vi "Parser signal by dbc.vi"(5 "ID array":i32[](array[numeric]) format="%.0x", 7 "NameShort":string[][](array[string])=[["Radar_AK_AMP", "Radar_AK_ANG", "Radar_AK_BSD_FLG", "Radar_AK_DST", "Radar_AK_ELE", "Radar_AK_EXST_PRB", "Radar_AK_Ego_Car_SPD", "Radar_AK_ID", "Radar_AK_LNG_ACC", "Radar_AK_MOV_FLG", "Radar_AK_RESERVE", "Radar_AK_SPD", "Radar_AK_Vx", "Radar_AK_Vy", "Radar_AK_Vz", "", "", "", "", "", "", "", "", "", "", "", "", "", "", ""], ["Radar_BK_2_AMP", "Radar_BK_2_ANG", "Radar_BK_2_DST", "Radar_BK_2_ELE", "Radar_BK_2_SPD", "Radar_BK_3_AMP", "Radar_BK_3_ANG", "Radar_BK_3_DST", "Radar_BK_3_ELE", "Radar_BK_3_SPD", "Radar_BK_4_AMP", "Radar_BK_4_ANG", "Radar_BK_4_DST", "Radar_BK_4_ELE", "Radar_BK_4_SPD", "Radar_BK_5_AMP", "Radar_BK_5_ANG", "Radar_BK_5_DST", "Radar_BK_5_ELE", "Radar_BK_5_SPD", "Radar_BK_6_AMP", "Radar_BK_6_ANG", "Radar_BK_6_DST", "Radar_BK_6_ELE", "Radar_BK_6_SPD", "Radar_BK_AMP", "Radar_BK_ANG", "Radar_BK_DST", "Radar_BK_ELE", "Radar_BK_SPD"], ["Radar_Header_Cdi_Number", "Radar_Header_Frame_Peroid", "Radar_Header_Frame_Type", "Radar_Header_Frame_id", "Radar_Header_Raw_Number", "Radar_Header_Track_Output_Number", "", "", "", "", "", "", "", "", "", "", "", "", "", "", "", "", "", "", "", "", "", "", "", ""], ["Radar_AK_Header_Number", "Radar_AK_Run_Time", "", "", "", "", "", "", "", "", "", "", "", "", "", "", "", "", "", "", "", "", "", "", "", "", "", "", "", ""]], 8 "error in (no error)":errorcluster caption="错误输入（无错误）", 9 "payload":u8[](array[numeric])=[140, 5, 0, 0, 0, 205, 218, 172, 202, 134, 212, 0, 0, 0, 0, 0, 20, 6, 0, 0, 0, 205, 214, 171, 199, 128, 12, 0, 0, 0, 0, 0, 107, 6, 0, 0, 0, 205, 86, 79, 7, 253, 54, 0, 0, 0, 0, 0, 0, 0, 0, 0, 0, 0, 0, 0, 0, 0, 0, 0, 0, 0, 0, 0] format="%.0x", 10 "ID":u32=1024 format="%.0x", 11 "Session":refnum<k21>[](array[refnum])) -> (0 "error out":errorcluster caption="错误输出", 1 "signal data":dbl[](array[numeric])=[1.0, -0.87, 0.0, 0.0, 0.27, 0.0, 0.0, 0.0, 0.0, -101.0, 14.200000000000001, 0.0, 27.32, -74.0, 0.0, 1.0, 0.25, 0.0, 0.0, 0.03, 0.0, 0.0, 0.0, 0.0, -101.0, 15.56, 0.0, 19.63, -82.0, 0.0, 0.0, 1.09, 0.0, 0.0, -0.12, 0.0, 0.0, 0.0, 0.0, -101.0, 16.43, 0.0, 18.71, -82.0, 0.0, 0.0, 0.0, 0.0, 0.0, 0.0, 0.0, 0.0, 0.0, 0.0, -255.0, 0.0, 0.0, 0.0, -255.0, 0.0] format="%.2f", 2 "Names":string[](array[string])=["LGU1_azAmb", "LGU1_azAngle", "LGU1_azAngleQly", "LGU1_elAmb", "LGU1_elAngle", "LGU1_elAngleQly", "LGU1_existProb", "LGU1_locPeerIdx", "LGU1_measStatus", "LGU1_noi", "LGU1_radDist", "LGU1_radVel", "LGU1_rcsEst", "LGU1_sigPwr", "LGU1_velQly", "LGU2_azAmb", "LGU2_azAngle", "LGU2_azAngleQly", "LGU2_elAmb", "LGU2_elAngle", "LGU2_elAngleQly", "LGU2_existProb", "LGU2_locPeerIdx", "LGU2_measStatus", "LGU2_noi", "LGU2_radDist", "LGU2_radVel", "LGU2_rcsEst", "LGU2_sigPwr", "LGU2_velQly", "LGU3_azAmb", "LGU3_azAngle", "LGU3_azAngleQly", "LGU3_elAmb", "LGU3_elAngle", "LGU3_elAngleQly", "LGU3_existProb", "LGU3_locPeerIdx", "LGU3_measStatus", "LGU3_noi", "LGU3_radDist", "LGU3_radVel", "LGU3_rcsEst", "LGU3_sigPwr", "LGU3_velQly", "LGU4_azAmb", "LGU4_azAngle", "LGU4_azAngleQly", "LGU4_elAmb", "LGU4_elAngle", "LGU4_elAngleQly", "LGU4_existProb", "LGU4_locPeerIdx", "LGU4_measStatus", "LGU4_noi", "LGU4_radDist", "LGU4_radVel", "LGU4_rcsEst", "LGU4_sigPwr", "LGU4_velQly"])   [LabVIEW 2024]
uses:
  <vilib>/xnet/xnet.llb/XNET Frame CAN.ctl
  <vilib>/xnet/xnet.llb/XNET Frame Type CAN.ctl
  <vilib>/xnet/xnet.llb/XNET Convert (Frame CAN to Signal).vi
panel:
  out "time":u32=4
  in  "frame data":T1[](array[typedef])=[{"timestamp"=timestamp(0 s since 1904-01-01), "payload"=[], "identifier"=0, "type"=16, "extended?"=FALSE, "echo?"=FALSE}] {"payload" format="%x"; "timestamp" format="%<%.7X\n%x>T"; "type" items=["CAN Data"=0, "CAN Remote"=1, "CAN Bus Error"=2, "CAN 2.0 Data"=8, "CAN FD Data"=16, "CAN FD+BRS Data"=24, "J1939 Data"=192, "Delay"=224, "Log Trigger"=225, "Start Trigger"=226]; "identifier" format="%x"}
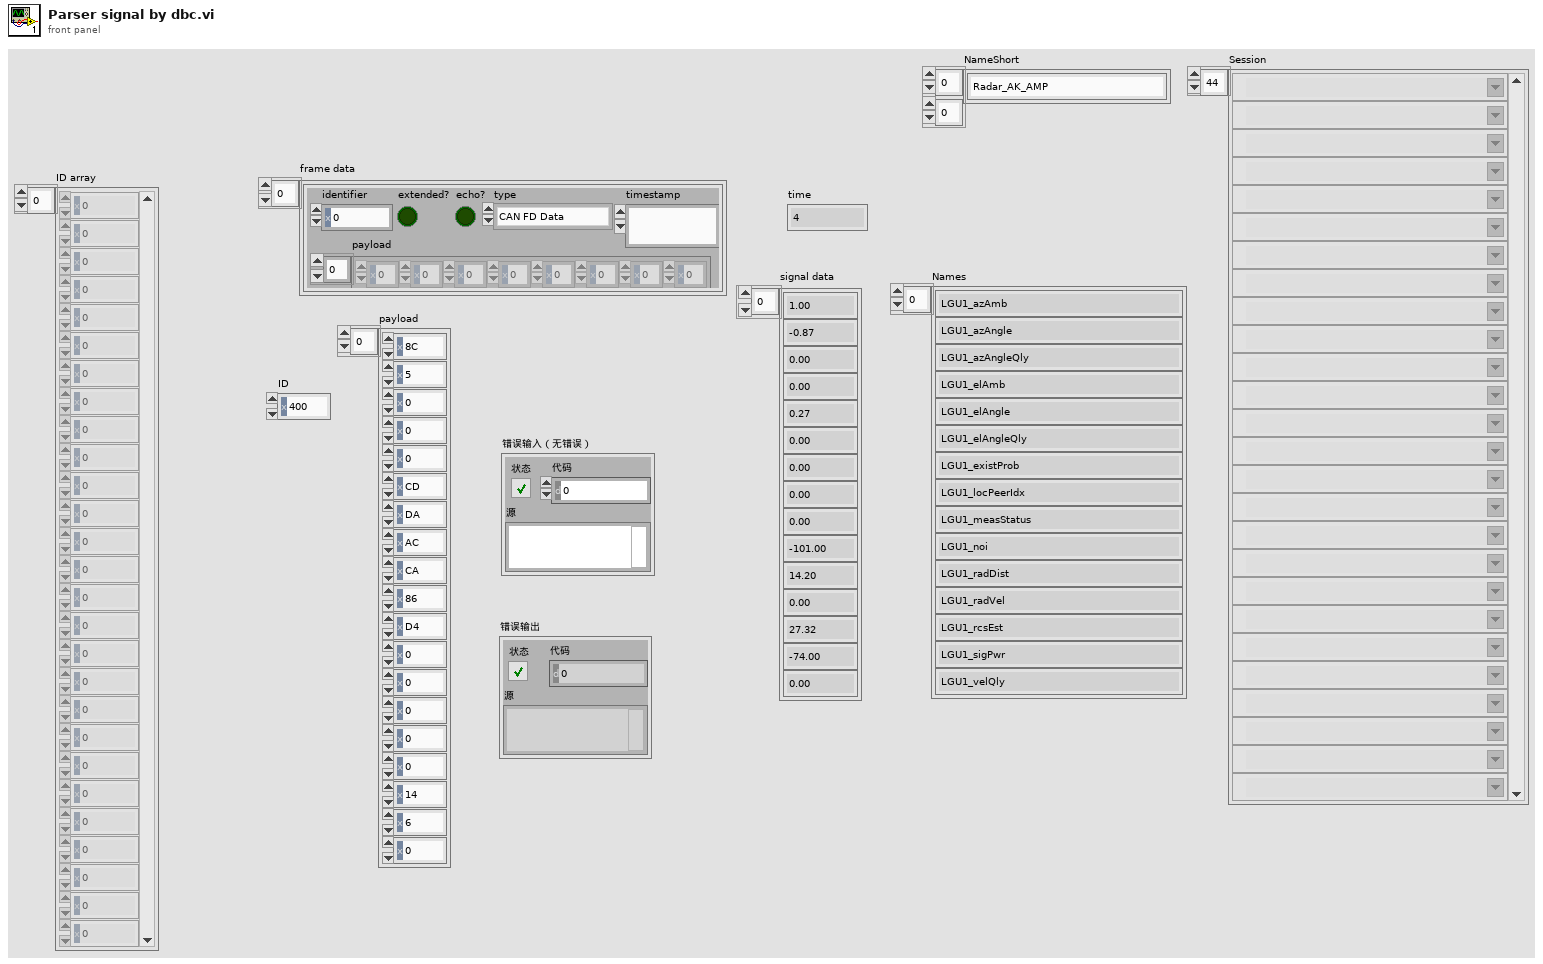
[diagram p1: front panel]
types:
  T1 = typedef "XNET Frame CAN.ctl" = cluster{"timestamp":timestamp, "payload":u8[], "identifier":u32, "type":T2, "extended?":bool, "echo?":bool}
  T2 = typedef "XNET Frame Type CAN.ctl" = u8
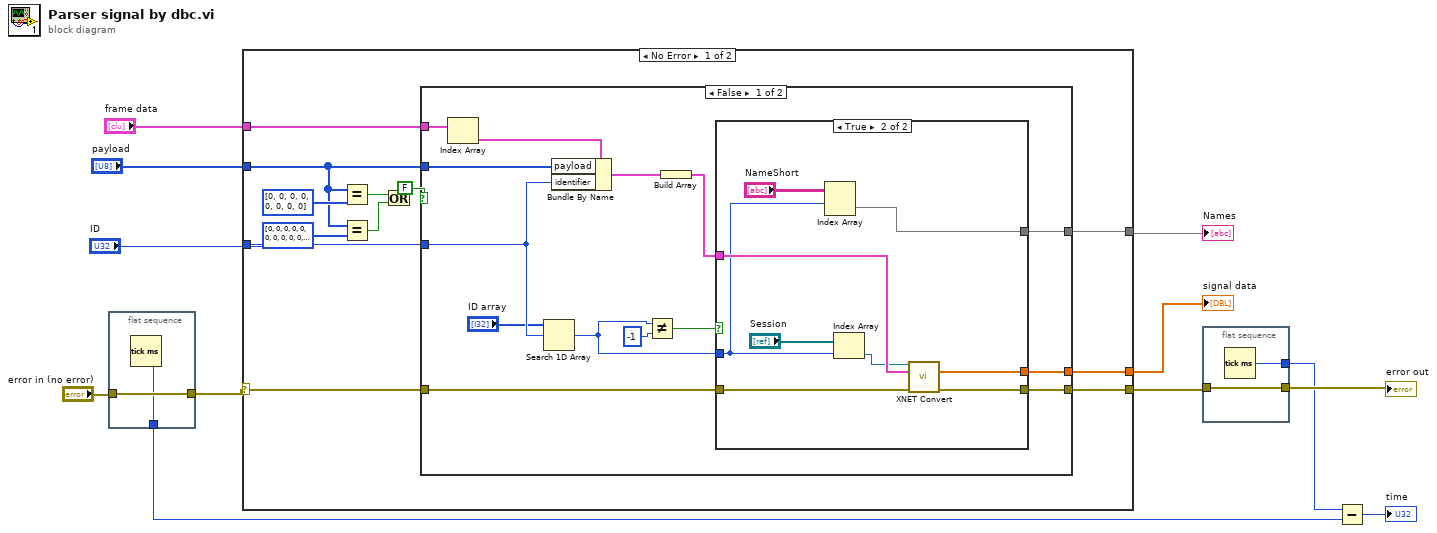
[diagram p0: block diagram]
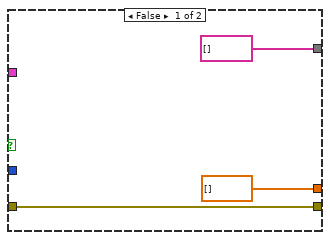
[diagram p2: hidden frame]
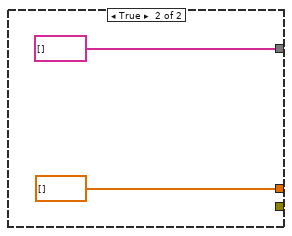
[diagram p3: hidden frame]
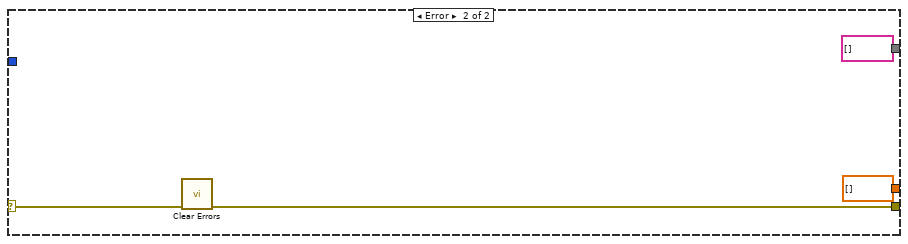
[diagram p4: hidden frame]
diagram:
  n1 = flat-sequence {
    tunnel: "error in (no error)" -> [w14]
    tunnel: [w14] -> w4
    tunnel: [w13] -> w2
    frame #0 {
      n2 = Tick Count (ms)() -> (millisecond timer value=w13:u32)
    }
  }
  n3 = case shown="No Error" w4 {
    selector: w4 -> [w22 w58]
    tunnel: [w26 dbl[] [] ("signal data")] -> w11
    tunnel: [w25 string[] [] ("Nameshort")] -> w12
    tunnel: "frame data" -> [w24 _]
    tunnel: "payload" -> [w19 _]
    tunnel: "ID" -> [w23 _]
    tunnel: [w21 w57] -> w7
    frame No Error {
      n4 = Equal?(x=w19, y=u8[] [0, 0, 0, 0, 0, 0, 0, 0] ("initialized array")) -> (x = y?=w17:bool)
      n5 = Equal?(x=w19, y=u8[] [0, 0, 0, 0, 0, 0, 0, 0, 0, 0, 0, 0, 0, 0, 0, 0, 0, 0, 0, 0, 0, 0, 0, 0, 0, 0, 0, 0, 0, 0, 0, 0, 0, 0, 0, 0, 0, 0, 0, 0, 0, 0, 0, 0, 0, 0, 0, 0, 0, 0, 0, 0, 0, 0, 0, 0, 0, 0, 0, 0, 0, 0, 0, 0] ("initialized array 2")) -> (x = y?=w16:bool)
      n6 = Or(x=w17, y=w16) -> ()  [unwired: 1 out]
      n7 = case shown="False" FALSE {
        tunnel: [w40 dbl[] [] ("signal data")] -> w26
        tunnel: [w39 string[] [] ("Nameshort")] -> w25
        tunnel: w24 -> [w38 _]
        tunnel: w23 -> [w30 _]
        tunnel: w22 -> [w37 _]
        tunnel: [w36 _] -> w21
        tunnel: w19 -> [w28 _]
        frame False {
          n8 = Index Array(array=w38) -> (element=w31:T1)  [unwired: 1 in]
          n9 = Search 1D Array(1D array="ID array", element=w30) -> (index of element=w35:i32)  [unwired: 1 in]
          n10 = Bundle By Name(cluster=w31, "payload"=w28, "identifier"=w30) -> (w33:T1)
          n11 = Not Equal?(x=w35, y=-1) -> (x != y?=w29:bool)
          n12 = Build Array(w33) -> (w34:T1[])
          n13 = case shown="True" w29 {
            tunnel: [dbl[] [] ("signal data") w52] -> w40
            tunnel: [string[] [] ("Nameshort") w51] -> w39
            tunnel: w34 -> [_ w50]
            tunnel: w35 -> [_ w48]
            tunnel: w37 -> [w43 w49]
            tunnel: [w43 w47] -> w36
            frame False {
            }
            frame True {
              n14 = Index Array(array="NameShort", index (row)=w48) -> (element=w51:string[])  [unwired: 1 in]
              n15 = Index Array(array="Session", index=w48) -> (element=w46:refnum<k21>)
              n16 = call-poly <vilib>:"XNET Convert.vi"("session in"=w46, "frame data"=w50, "error in (no error)"=w49) -> ("signal data"=w52:dbl[], "error out"=w47:errorcluster)  [unwired: 10 in, 1 out]
            }
          }
        }
        frame True {
        }
      }
    }
    frame Error {
      n17 = call <vilib>:"Clear Errors.vi"("error in (no error)"=w58) -> ("error out"=w57:errorcluster)  [unwired: 5 in, 1 out]
    }
  }
  "signal data" <- w11
  "Names" <- w12
  n18 = flat-sequence {
    tunnel: w7 -> [w60]
    tunnel: [w60] -> w6
    tunnel: [w59] -> w3
    frame #0 {
      n19 = Tick Count (ms)() -> (millisecond timer value=w59:u32)
    }
  }
  n20 = Subtract(x=w3, y=w2) -> (x-y=→"time":u32)
  "error out" <- w6
